vi "DVT_EXTERNAL.vi"(3 "Ch_Status?":bool=TRUE, 4 "ms":u32=10, 5 "write buffer":string, 6 "VISA resource name":refnum<visa-resource-name>="COM13") -> (0 "error out":errorcluster, 1 "Boolean array":bool[](array[boolean]), 2 "VISA resource name out":refnum<visa-resource-name>)   [LabVIEW 2019]
panel:
  # "Command \t\n\nAction\ndec \thex normal\n56 \t38 \t      8         Get serial number - returns 8 bytes of ASCII that form the unique serial number for module, I.E \"00001543\"\n90 \t5A \t      Z        Get software version - returns 2 bytes, the first being the Module ID which is 8, followed by the software version\n91 \t5B \t       [       Get relay states - sends a single byte back to the controller, bit high meaning the corresponding relay is powered\n92 \t5C \t        \\      Set relay states - the next single byte will set all relays states, All on = 255 (11111111) All off = 0\n100 \t64        d     \tAll relays on\n101 \t65        e     \tTurn relay 1 on\n102 \t66        f      Turn relay 2 on\n103 \t67       g      \tTurn relay 3 on\n104 \t68       h      \tTurn relay 4 on\n105 \t69 \t     i       Turn relay 5 on\n106 \t6A \t   j        Turn relay 6 on\n107 \t6B \t  k         Turn relay 7 on\n108 \t6C \t  l         Turn relay 8 on\n110 \t6E \t  n          All relays off\n111 \t6F     o        \tTurn relay 1 off\n112 \t70 \t   p         Turn relay 2 off\n113 \t71     q        \tTurn relay 3 off\n114 \t72 \t   r         Turn relay 4 off\n115 \t73     s        \tTurn relay 5 off\n116 \t74 \t   t         Turn relay 6 off\n117 \t75 \t   u         Turn relay 7 off\n118 \t76     v        \tTurn relay 8 off"
  # "h-r    Mixer ON/OFF\ni-s     Halogen\nj-t     Shutter\nk-u   Deuterium\nl-v    Power Strip"
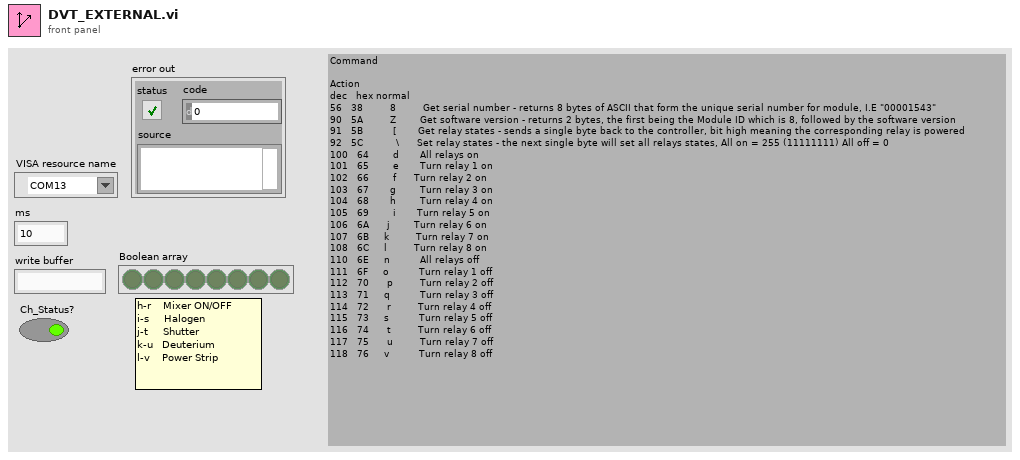
[diagram p1: front panel]
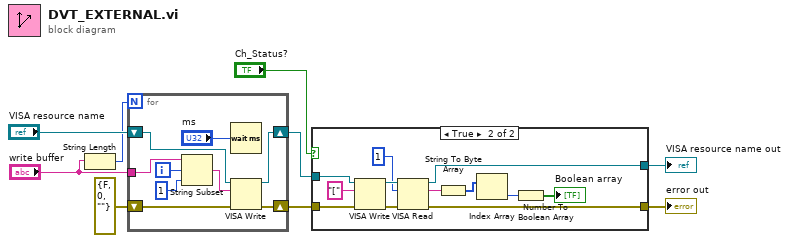
[diagram p0: block diagram]
diagram:
  n1 = String Length(string="write buffer") -> (length=w3:i32)
  n2 = for {
    N: w3 -> [_]
    tunnel: "write buffer" -> [w13]
    shift-right: [w16] -> w7
    shift-left: "VISA resource name" -> [w18]
    shift-right: [w17] -> w8
    shift-left: errorcluster {"status"=FALSE, "code"=0, "source"=""} ("error out") -> [w11]
    i -> [w15]
    n3 = String Subset(string=w13, offset (0)=w15, length (rest)=1 ("length (rest)")) -> (substring=w12:string)
    n4 = Wait (ms)(milliseconds to wait="ms") -> ()  [unwired: 1 out]
    n5 = VISA Write(VISA resource name=w18, write buffer=w12, error in (no error)=w11) -> (VISA resource name out=w16:refnum<visa-resource-name>, error out=w17:errorcluster)  [unwired: 1 out]
  }
  n6 = case shown="True" "Ch_Status?" {
    tunnel: w8 -> [w19 w32]
    tunnel: w7 -> [w20 w31]
    tunnel: [w20 w26] -> w6
    tunnel: [w19 w25] -> w5
    frame False {
    }
    frame True {
      n7 = VISA Write(VISA resource name=w31, write buffer="[" ("write buffer 2"), error in (no error)=w32) -> (VISA resource name out=w29:refnum<visa-resource-name>, error out=w28:errorcluster)  [unwired: 1 out]
      n8 = VISA Read(VISA resource name=w29, byte count=u32 1, error in (no error)=w28) -> (VISA resource name out=w26:refnum<visa-resource-name>, read buffer=w23:string, error out=w25:errorcluster)  [unwired: 1 out]
      n9 = String To Byte Array(string=w23) -> (unsigned byte array=w22:u8[])
      n10 = Index Array(array=w22) -> (element=w21:u8)  [unwired: 1 in]
      n11 = Number To Boolean Array(number=w21) -> (Boolean array=→"Boolean array":bool[])
    }
  }
  "VISA resource name out" <- w6
  "error out" <- w5
